vi "TCP Data Stream PC (by ref).vi"(0 "RT IP Address":string, 5 "Error IN":errorcluster, 6 "Mode":T1, 9 "TCP Stream Ref":refnum<vi>) -> (14 "Data OUT":dbl[][](array[numeric]), 15 "New Data?":bool, 16 "Connected?":bool, 19 "Error OUT":errorcluster)   [LabVIEW 2019]
uses:
  Type Defs and Controls/TCP Data Stream Mode (PC).ctl
  Type Defs and Controls/TCP Data Stream Mode.ctl
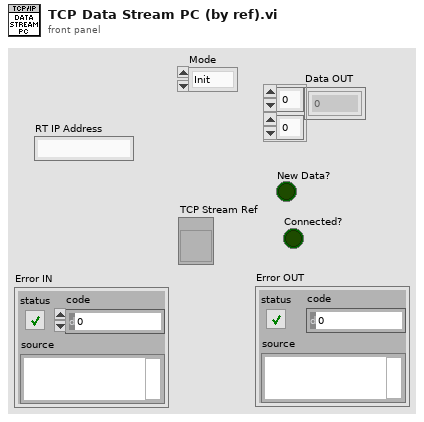
[diagram p1: front panel]
types:
  T1 = typedef "TCP Data Stream Mode (PC).ctl" = enum16{"Init", "Read Data", "Close"}
  T2 = typedef "TCP Data Stream Mode.ctl" = enum16{"Init RT", "Init PC", "Connect RT", "Connect PC", "Write Data", "Read Data", "Close"}
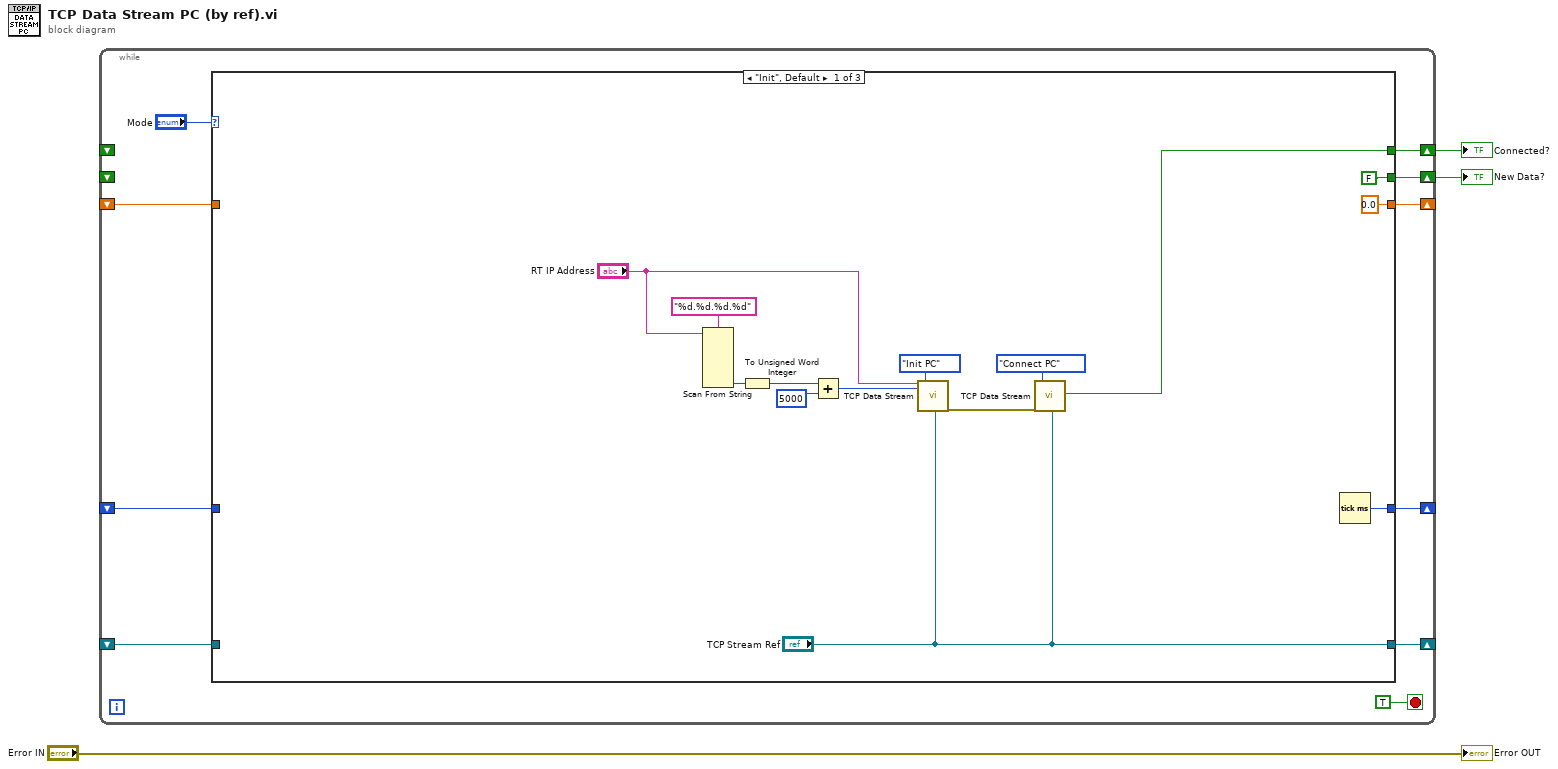
[diagram p0: block diagram]
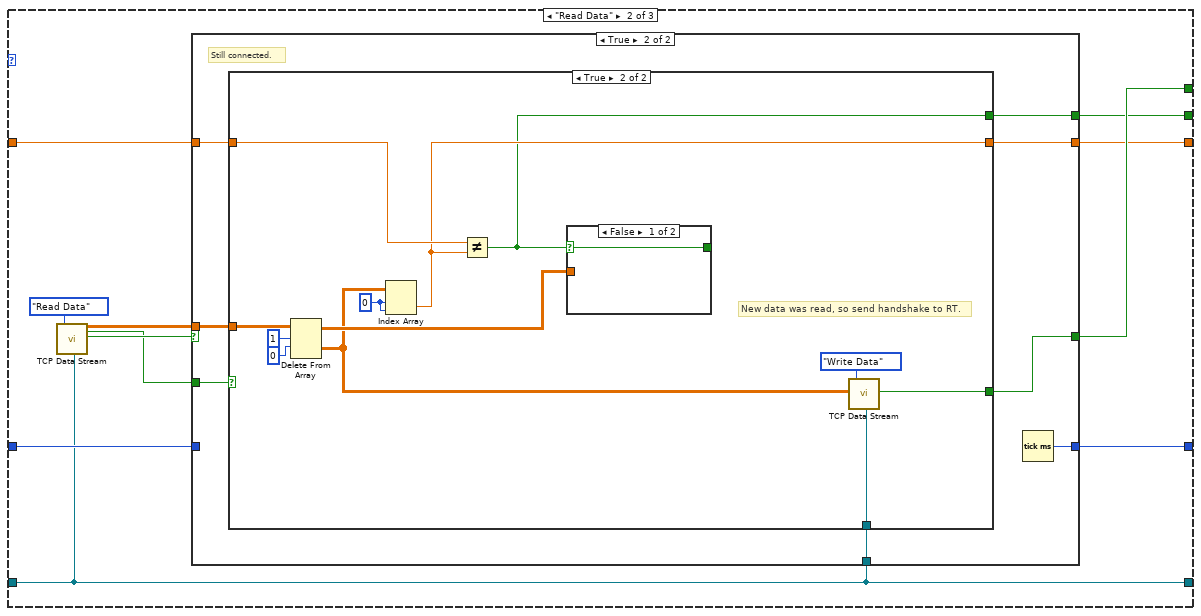
[diagram p2: hidden frame]
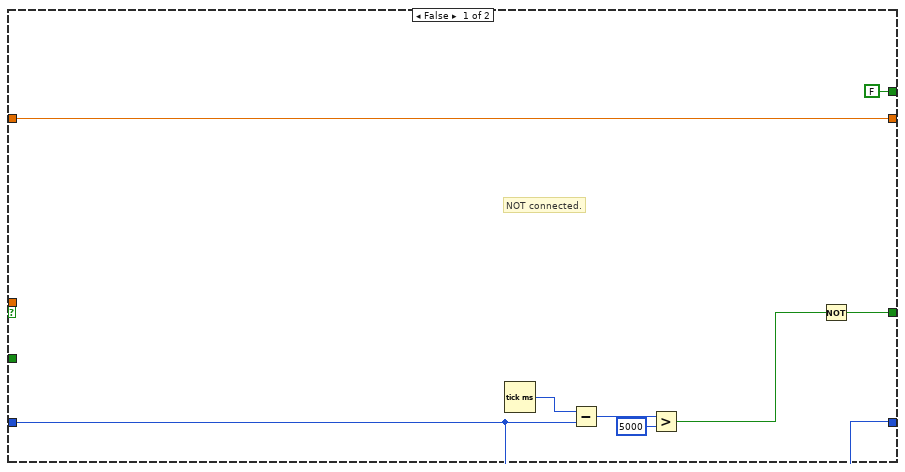
[diagram p3: hidden frame]
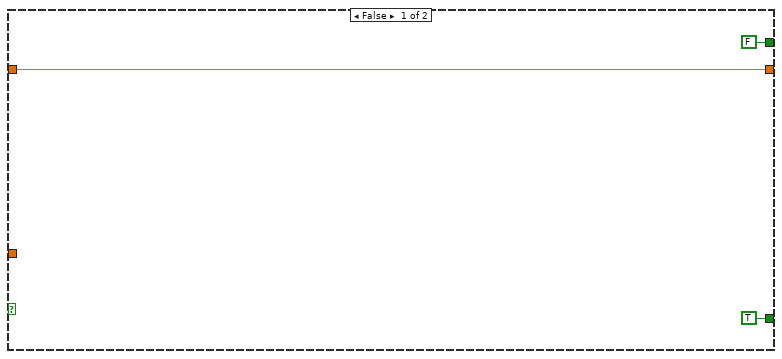
[diagram p4: hidden frame]
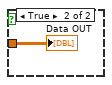
[diagram p5: hidden frame]
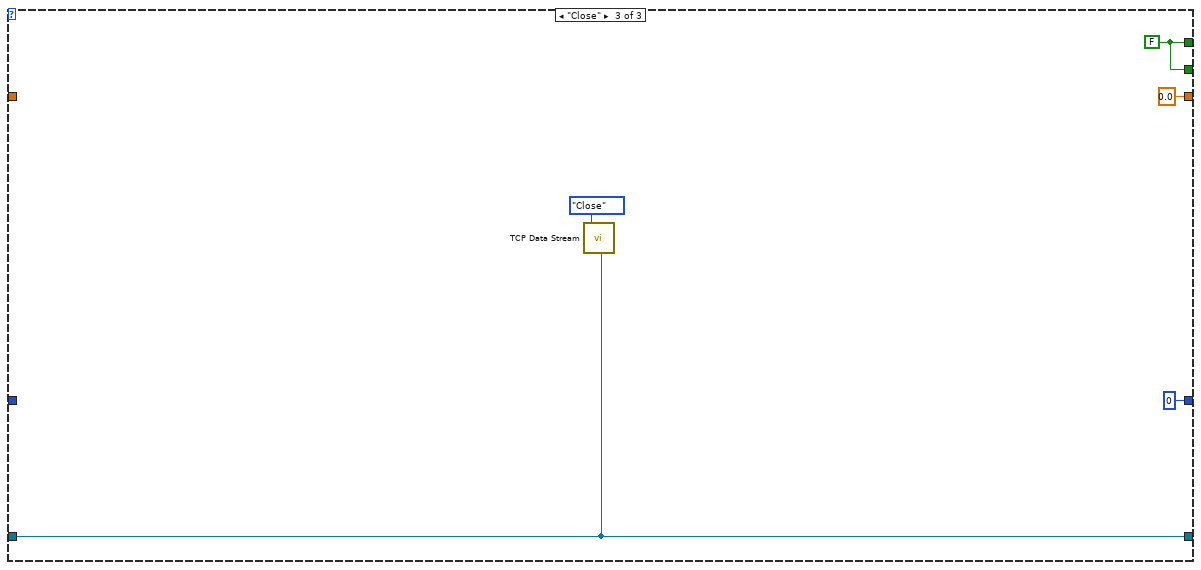
[diagram p6: hidden frame]
diagram:
  n1 = while {
    shift-right: [w11] -> w2
    shift-left: _ -> [_]
    shift-right: [w10] -> w1
    shift-left: _ -> [_]
    shift-right: [w9] -> _
    shift-left: _ -> [w8]
    shift-right: [w7] -> _
    shift-left: _ -> [w6]
    shift-right: [w5] -> _
    shift-left: _ -> [w4]
    stop <- TRUE stop-if-true
    n2 = case shown="\"Init\", Default" "Mode" {
      tunnel: [w15 w36 w76] -> w11
      tunnel: [FALSE ("Connected?") w29 w76] -> w10
      tunnel: [w17 w34 u32 0 ("millisecond timer value")] -> w9
      tunnel: w8 -> [_ w35 _]
      tunnel: [0.0 w30 0.0] -> w7
      tunnel: w6 -> [_ w31 _]
      tunnel: ["TCP Stream Ref" w28 w72] -> w5
      tunnel: w4 -> [_ w28 w72]
      frame "Init", Default {
        n3 = Scan From String(format string="%d.%d.%d.%d", input string="RT IP Address") -> (output 4=w26:i32)  [unwired: 9 in, 3 out]
        n4 = To Unsigned Word Integer(number=w26) -> (unsigned 16bit integer=w24:u16)
        n5 = Add(x=w24, y=u16 5000 ("Port")) -> (x+y=w18:u16)
        n6 = call "TCP Data Stream.vi"("Address"="RT IP Address", "Port"=w18, "Mode"=TCP_Data_Stream_Mode."Init PC", "TCP Stream Ref"="TCP Stream Ref") -> ("Error OUT"=w19:errorcluster)  [unwired: 11 in, 4 out]
        n7 = call "TCP Data Stream.vi"("Error IN"=w19, "Mode"=TCP_Data_Stream_Mode."Connect PC", "TCP Stream Ref"="TCP Stream Ref") -> ("Connected?"=w15:bool)  [unwired: 12 in, 4 out]
        n8 = Tick Count (ms)() -> (millisecond timer value=w17:u32)
      }
      frame "Read Data" {
        n9 = call "TCP Data Stream.vi"("Mode"=TCP_Data_Stream_Mode."Read Data", "TCP Stream Ref"=w28) -> ("Data OUT"=w32:dbl[][], "New Data?"=w33:bool, "Connected?"=w37:bool)  [unwired: 13 in, 2 out]
        n10 = case shown="True" w37 {
          tunnel: w33 -> [_ w54]
          tunnel: [w43 w53] -> w36
          tunnel: w35 -> [w41 _]
          tunnel: [w41 w52] -> w34
          tunnel: w32 -> [_ w51]
          tunnel: w31 -> [w40 w50]
          tunnel: [w40 w49] -> w30
          tunnel: [FALSE w48] -> w29
          tunnel: w28 -> [_ w47]
          frame False {
            # "NOT connected."
            n11 = Tick Count (ms)() -> (millisecond timer value=w42:u32)
            n12 = Subtract(x=w42, y=w41) -> (x-y=w46:u32)
            n13 = Greater?(x=w46, y=u32 5000) -> (0:w44:bool)
            n14 = Not(x=w44) -> (.not. x?=w43:bool)
          }
          frame True {
            # "Still connected."
            n15 = case shown="True" w54 {
              tunnel: [TRUE ("Connected?") w69] -> w53
              tunnel: w51 -> [_ w64]
              tunnel: w50 -> [w56 w62]
              tunnel: [w56 w61] -> w49
              tunnel: [FALSE w60] -> w48
              tunnel: w47 -> [_ w58]
              frame False {
              }
              frame True {
                w65 = 0 ("index (row)")
                # "New data was read, so send handshake to RT."
                n16 = Delete From Array(array=w64, length=1, index (row)=0) -> (deleted portion=w63:dbl[][], array with subset deleted=w68:dbl[][])  [unwired: 1 in]
                n17 = Index Array(array=w63, index (row)=w65, index (col)=w65) -> (element=w61:dbl)
                n18 = Not Equal?(x=w62, y=w61) -> (x != y?=w60:bool)
                n19 = case shown="False" w60 {
                  selector: w60 -> [w70 _]
                  tunnel: w68 -> [_ w71]
                  tunnel: [w70 _] -> _
                  frame False {
                  }
                  frame True {
                    "Data OUT" <- w71
                  }
                }
                n20 = call "TCP Data Stream.vi"("Data IN"=w63, "Mode"=TCP_Data_Stream_Mode."Write Data", "TCP Stream Ref"=w58) -> ("Connected?"=w69:bool)  [unwired: 12 in, 4 out]
              }
            }
            n21 = Tick Count (ms)() -> (millisecond timer value=w52:u32)
          }
        }
      }
      frame "Close" {
        w76 = FALSE ("Connected?")
        n22 = call "TCP Data Stream.vi"("Mode"=TCP_Data_Stream_Mode."Close", "TCP Stream Ref"=w72) -> ()  [unwired: 13 in, 5 out]
      }
    }
  }
  "Connected?" <- w2
  "New Data?" <- w1
  "Error OUT" <- "Error IN"
